vi "RT Main v0.1.vi"() -> ()   [LabVIEW 2017]
uses:
  support/Controls/All Inputs.ctl
  support/Controls/Index Details.ctl
  Controls/Auto Delays.ctl
  Global Variables/FPGA GV.vi
  <vilib>/Utility/error.llb/Error Cluster From Error Code.vi
  <vilib>/rvi/errors/niLvFpgaAdjustHostInterfaceError.vi
  Global Variables/Network Globals.vi
  Global Variables/RT GV.vi
  support/Message Queue/Enqueue Message (Single).vi
  <vilib>/FPGAPlugInAG/Dynamic/niLvFpga_Close_Dynamic.vi
  <vilib>/rvi/interface/nirviReadWriteControl/nirviReadWriteControl.xnode
  Controls/FPGA Ref.ctl
  <vilib>/rvi/interface/nirviCloseFPGA/nirviCloseFPGA.xnode
  support/Message Queue/Message Queue.lvlib
  NiFpgaLv.dll
  <vilib>/rvi/interface/Simulation/niFpgaSimulationCallBeginRW.vi
panel:
  out "error out":errorcluster
  out "Wrong Message":string
  in  "Stop Button":bool
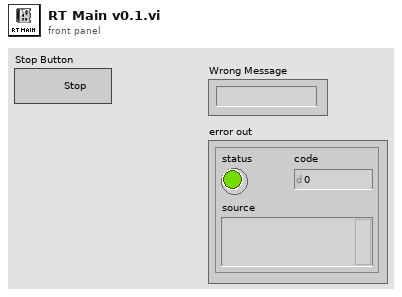
[diagram p1: front panel]
types:
  T1 = typedef "FPGA Ref.ctl" = refnum<k20>
  T2 = cluster{"TL_Red":bool, "TL_Orange":bool, "TL_Green":bool, "TL_Buzzer":bool, "SOL_Index_Rotary_CW":bool, "SOL_Index_CNVR_Rotary_CCW":bool, "SOL_Index_CNVR_Stopper_Rear":bool, "SOL_Index_CNVR_Output _Separator _Rear":bool, "Bowl  Feeder_ ON":bool, "Pump_CNVR_Motor _ON":bool, "SOL_Gating_CYL_Rear":bool, "SOL_Tube_Feed_Agitatator":bool, "SOL_Tube_Feed_Gating_CYL":bool, "SOL_Insertion _CYL":bool, "SOL_Insertion_Clamp_CYL":bool, "SOL_Cutting_CYL":bool, "SOL_Cutting_Clamp_CYL":bool, "SOL_Insertion_Air_Nozzle":bool, "SOL_Measurement_CYL":bool, "SOL_Measure_Clamp_CYL":bool, "SOL_Rejection CYL_1":bool, "SOL_Rejection CYL_2":bool, "SOL_Rejection CYL_3":bool, "SOL_Rejection CYL_4":bool, "DO1.24":bool, "DO1.25":bool, "DO1.26":bool, "DO1.27":bool, "DO1.28":bool, "DO1.29":bool, "DO1.30":bool, "DO1.31":bool}
  T3 = typedef "All Inputs.ctl" = cluster{"DI 1":cluster{"Machine_ON":bool, "E_stop ":bool, "SW_Pressure":bool, "SW_Start ":bool, "SW_Reset":bool, "SW_Stop":bool, "SW_Door":bool, "RS_Index_Rotary_CW":bool, "RS_Index_Rotary_CCW":bool, "RS_Index_Stopper _Rear":bool, "RS_Index_Output_Separator_Rear":bool, "PES_Index_Pallet_Sensor":bool, "PES_Index_Output_Part Sensor":bool, "ICS_BF_Low_Level_1":bool, "ICS_BF_Low_Level_2":bool, "ICS_BF_Pump_CNVR_Full_1":bool, "ICS_BF_Pump_CNVR_Full_2":bool, "ICS_BF_Pump_CNVR_Full_3":bool, "ICS_BF_Pump_CNVR_Full_4":bool, "PES_PC_Pump Presence_1":bool, "PES_PC_Pump Presence_2":bool, "PES_PC_Pump Presence_3":bool, "PES_PC_Pump Presence_4":bool, "RS_Gating_Rear":bool, "PES_Pump_Interference":bool, "PES_TF_Low_Level":bool, "PES_Tube Presence_1":bool, "PES_Tube Presence_2":bool, "PES_Tube Presence_3":bool, "PES_Tube Presence_4":bool, "DI1.30":bool, "DI1.31":bool}, "DI 2":cluster{"RS_Agitatator_1_Rear ":bool, "RS_Agitatator_2_Rear ":bool, "RS_Gating CYL_Rear":bool, "RS_Insertion_1_Rear":bool, "RS_Insertion_1_Front":bool, "RS_Insertion _2_Rear":bool, "RS_Insertion _2_Front":bool, "RS_Insertion _3_Rear":bool, "RS_Insertion _3_Front":bool, "RS_Insertion _4_Rear":bool, "RS_Insertion _4_Front":bool, "RS_Insertion_Clamp_Rear":bool, "RS_Cutting_Rear":bool, "RS_Cutting_Clamp _Rear":bool, "RS_Measurement_1_Rear":bool, "RS_Measurement_2_Rear":bool, "RS_Measurement_3_Rear":bool, "RS_Measurement_4_Rear":bool, "RS_Measure_Clamp_Rear":bool, "RS_Rejection_1_Rear":bool, "RS_Rejection_2_Rear":bool, "RS_Rejection_3_Rear":bool, "RS_Rejection_4_Rear":bool, "DI2.23":bool, "DI2.24":bool, "DI2.25":bool, "DI2.26":bool, "DI2.27":bool, "DI2.28":bool, "DI2.29":bool, "DI2.30":bool, "DI2.31":bool}, "IAS 1":dbl, "IAS 2":dbl, "IAS 3":dbl, "IAS 4":dbl, "DO 1":cluster{"TL_Red":bool, "TL_Orange":bool, "TL_Green":bool, "TL_Buzzer":bool, "SOL_Index_Rotary_CW":bool, "SOL_Index_CNVR_Rotary_CCW":bool, "SOL_Index_CNVR_Stopper_Rear":bool, "SOL_Index_CNVR_Output _Separator _Rear":bool, "Bowl  Feeder_ ON":bool, "Pump_CNVR_Motor _ON":bool, "SOL_Gating_CYL_Rear":bool, "SOL_Tube_Feed_Agitatator":bool, "SOL_Tube_Feed_Gating_CYL":bool, "SOL_Insertion _CYL":bool, "SOL_Insertion_Clamp_CYL":bool, "SOL_Cutting_CYL":bool, "SOL_Cutting_Clamp_CYL":bool, "SOL_Insertion_Air_Nozzle":bool, "SOL_Measurement_CYL":bool, "SOL_Measure_Clamp_CYL":bool, "SOL_Rejection CYL_1":bool, "SOL_Rejection CYL_2":bool, "SOL_Rejection CYL_3":bool, "SOL_Rejection CYL_4":bool, "DO1.24":bool, "DO1.25":bool, "DO1.26":bool, "DO1.27":bool, "DO1.28":bool, "DO1.29":bool, "DO1.30":bool, "DO1.31":bool}}
  T4 = typedef "Index Details.ctl" = cluster{"Time (ms)":u32, "Waveform Graph":i16[]}
  T5 = typedef "Auto Delays.ctl" = cluster{"TF Delays":u32[], "Insertion Delays":u32[], "Cutting Delays":u32[]}
  T6 = cluster{"Machine_ON":bool, "E_stop ":bool, "SW_Pressure":bool, "SW_Start ":bool, "SW_Reset":bool, "SW_Stop":bool, "SW_Door":bool, "RS_Index_Rotary_CW":bool, "RS_Index_Rotary_CCW":bool, "RS_Index_Stopper _Rear":bool, "RS_Index_Output_Separator_Rear":bool, "PES_Index_Pallet_Sensor":bool, "PES_Index_Output_Part Sensor":bool, "ICS_BF_Low_Level_1":bool, "ICS_BF_Low_Level_2":bool, "ICS_BF_Pump_CNVR_Full_1":bool, "ICS_BF_Pump_CNVR_Full_2":bool, "ICS_BF_Pump_CNVR_Full_3":bool, "ICS_BF_Pump_CNVR_Full_4":bool, "PES_PC_Pump Presence_1":bool, "PES_PC_Pump Presence_2":bool, "PES_PC_Pump Presence_3":bool, "PES_PC_Pump Presence_4":bool, "RS_Gating_Rear":bool, "PES_Pump_Interference":bool, "PES_TF_Low_Level":bool, "PES_Tube Presence_1":bool, "PES_Tube Presence_2":bool, "PES_Tube Presence_3":bool, "PES_Tube Presence_4":bool, "DI1.30":bool, "DI1.31":bool}
  T7 = cluster{"RS_Agitatator_1_Rear ":bool, "RS_Agitatator_2_Rear ":bool, "RS_Gating CYL_Rear":bool, "RS_Insertion_1_Rear":bool, "RS_Insertion_1_Front":bool, "RS_Insertion _2_Rear":bool, "RS_Insertion _2_Front":bool, "RS_Insertion _3_Rear":bool, "RS_Insertion _3_Front":bool, "RS_Insertion _4_Rear":bool, "RS_Insertion _4_Front":bool, "RS_Insertion_Clamp_Rear":bool, "RS_Cutting_Rear":bool, "RS_Cutting_Clamp _Rear":bool, "RS_Measurement_1_Rear":bool, "RS_Measurement_2_Rear":bool, "RS_Measurement_3_Rear":bool, "RS_Measurement_4_Rear":bool, "RS_Measure_Clamp_Rear":bool, "RS_Rejection_1_Rear":bool, "RS_Rejection_2_Rear":bool, "RS_Rejection_3_Rear":bool, "RS_Rejection_4_Rear":bool, "DI2.23":bool, "DI2.24":bool, "DI2.25":bool, "DI2.26":bool, "DI2.27":bool, "DI2.28":bool, "DI2.29":bool, "DI2.30":bool, "DI2.31":bool}
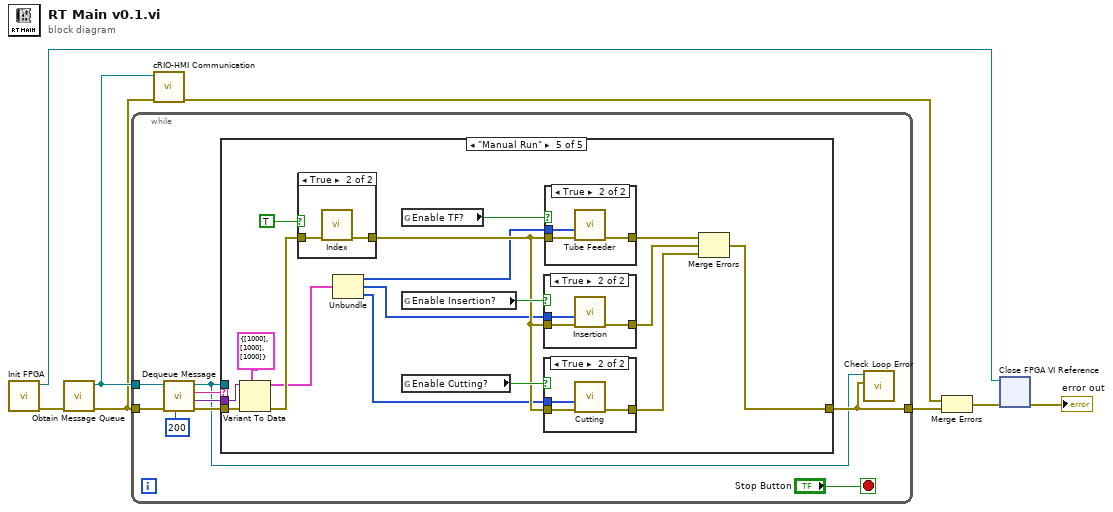
[diagram p0: block diagram]
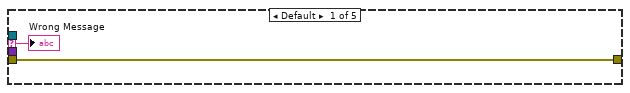
[diagram p2: hidden frame]
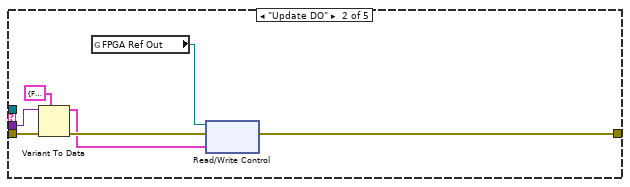
[diagram p3: hidden frame]
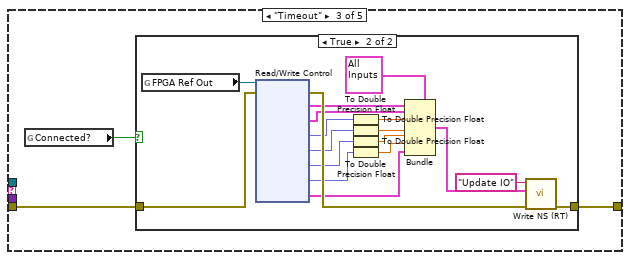
[diagram p4: hidden frame]
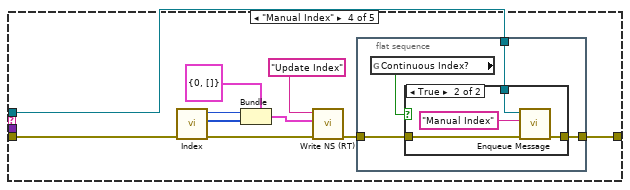
[diagram p6: hidden frame]
diagram:
  n1 = call "Init FPGA.vi"() -> ("error out"=w8:errorcluster, "FPGA Ref Out"=w2:T1)  [unwired: 10 in]
  n2 = call "Obtain Message Queue.vi"("error in (no error)"=w8) -> ("error out"=w1:errorcluster, "Message Queue"=w7:refnum<queue>)  [unwired: 9 in]
  n3 = while {
    tunnel: w1 -> [w16]
    tunnel: w7 -> [w15]
    tunnel: [w11] -> w6
    stop <- "Stop Button" stop-if-true
    n4 = call "Dequeue Message.vi"("timeout"=200, "error in (no error)"=w16, "Message Queue"=w15) -> ("error out"=w14:errorcluster, "Message Data"=w12:variant, "Message"=w13:string, "dup Message Queue"=w10:refnum<queue>)  [unwired: 5 in]
    n5 = case shown="\"Manual Run\"" w13 {
      selector: w13 -> [w19 _ _ _ _]
      tunnel: w14 -> [w18 w26 w28 w58 w75]
      tunnel: w10 -> [_ _ _ w50 _]
      tunnel: w12 -> [_ w25 _ _ w68]
      tunnel: [w18 w21 w29 w51 w76] -> w11
      frame Default {
        "Wrong Message" <- w19
      }
      frame "Update DO" {
        n6 = Variant To Data(error in=w26, type=T2 {"TL_Red"=FALSE, "TL_Orange"=FALSE, "TL_Green"=FALSE, "TL_Buzzer"=FALSE, "SOL_Index_Rotary_CW"=FALSE, "SOL_Index_CNVR_Rotary_CCW"=FALSE, "SOL_Index_CNVR_Stopper_Rear"=FALSE, "SOL_Index_CNVR_Output _Separator _Rear"=FALSE, "Bowl  Feeder_ ON"=FALSE, "Pump_CNVR_Motor _ON"=FALSE, "SOL_Gating_CYL_Rear"=FALSE, "SOL_Tube_Feed_Agitatator"=FALSE, "SOL_Tube_Feed_Gating_CYL"=FALSE, "SOL_Insertion _CYL"=FALSE, "SOL_Insertion_Clamp_CYL"=FALSE, "SOL_Cutting_CYL"=FALSE, "SOL_Cutting_Clamp_CYL"=FALSE, "SOL_Insertion_Air_Nozzle"=FALSE, "SOL_Measurement_CYL"=FALSE, "SOL_Measure_Clamp_CYL"=FALSE, "SOL_Rejection CYL_1"=FALSE, "SOL_Rejection CYL_2"=FALSE, "SOL_Rejection CYL_3"=FALSE, "SOL_Rejection CYL_4"=FALSE, "DO1.24"=FALSE, "DO1.25"=FALSE, "DO1.26"=FALSE, "DO1.27"=FALSE, "DO1.28"=FALSE, "DO1.29"=FALSE, "DO1.30"=FALSE, "DO1.31"=FALSE} ("DO 1"), Variant=w25) -> (data=w20:T2, error out=w22:errorcluster)
        n7 = global read "FPGA GV.vi" "FPGA Ref Out"() -> (w23:T1)
        n8 = xnode "Read/Write Control"("FPGA VI Reference In"=w23, "error in"=w22, "DO 1"=w20) -> ("error out"=w21:errorcluster)  [unwired: 1 out]
      }
      frame "Timeout" {
        n9 = global read "Network Globals.vi" "Connected?"() -> (w27:bool)
        n10 = case shown="True" w27 {
          tunnel: [w30 w47] -> w29
          tunnel: w28 -> [w30 w45]
          frame False {
          }
          frame True {
            n11 = global read "FPGA GV.vi" "FPGA Ref Out"() -> (w46:T1)
            n12 = xnode "Read/Write Control"("FPGA VI Reference In"=w46, "error in"=w45) -> ("error out"=w44:errorcluster, "DI 1"=w43:T6, "DI 2"=w42:T7, "AI0"=w41:fxp<+/-,27,6>, "AI1"=w36:fxp<+/-,27,6>, "AI2"=w35:fxp<+/-,27,6>, "AI3"=w34:fxp<+/-,27,6>, "DO 1"=w31:T2)  [unwired: 1 out]
            n13 = To Double Precision Float(number=w41) -> (double precision float=w40:dbl)
            n14 = To Double Precision Float(number=w36) -> (double precision float=w39:dbl)
            n15 = To Double Precision Float(number=w35) -> (double precision float=w38:dbl)
            n16 = To Double Precision Float(number=w34) -> (double precision float=w37:dbl)
            n17 = Bundle(cluster=T3 {"DI 1"={"Machine_ON"=FALSE, "E_stop "=FALSE, "SW_Pressure"=FALSE, "SW_Start "=FALSE, "SW_Reset"=FALSE, "SW_Stop"=FALSE, "SW_Door"=FALSE, "RS_Index_Rotary_CW"=FALSE, "RS_Index_Rotary_CCW"=FALSE, "RS_Index_Stopper _Rear"=FALSE, "RS_Index_Output_Separator_Rear"=FALSE, "PES_Index_Pallet_Sensor"=FALSE, "PES_Index_Output_Part Sensor"=FALSE, "ICS_BF_Low_Level_1"=FALSE, "ICS_BF_Low_Level_2"=FALSE, "ICS_BF_Pump_CNVR_Full_1"=FALSE, "ICS_BF_Pump_CNVR_Full_2"=FALSE, "ICS_BF_Pump_CNVR_Full_3"=FALSE, "ICS_BF_Pump_CNVR_Full_4"=FALSE, "PES_PC_Pump Presence_1"=FALSE, "PES_PC_Pump Presence_2"=FALSE, "PES_PC_Pump Presence_3"=FALSE, "PES_PC_Pump Presence_4"=FALSE, "RS_Gating_Rear"=FALSE, "PES_Pump_Interference"=FALSE, "PES_TF_Low_Level"=FALSE, "PES_Tube Presence_1"=FALSE, "PES_Tube Presence_2"=FALSE, "PES_Tube Presence_3"=FALSE, "PES_Tube Presence_4"=FALSE, "DI1.30"=FALSE, "DI1.31"=FALSE}, "DI 2"={"RS_Agitatator_1_Rear "=FALSE, "RS_Agitatator_2_Rear "=FALSE, "RS_Gating CYL_Rear"=FALSE, "RS_Insertion_1_Rear"=FALSE, "RS_Insertion_1_Front"=FALSE, "RS_Insertion _2_Rear"=FALSE, "RS_Insertion _2_Front"=FALSE, "RS_Insertion _3_Rear"=FALSE, "RS_Insertion _3_Front"=FALSE, "RS_Insertion _4_Rear"=FALSE, "RS_Insertion _4_Front"=FALSE, "RS_Insertion_Clamp_Rear"=FALSE, "RS_Cutting_Rear"=FALSE, "RS_Cutting_Clamp _Rear"=FALSE, "RS_Measurement_1_Rear"=FALSE, "RS_Measurement_2_Rear"=FALSE, "RS_Measurement_3_Rear"=FALSE, "RS_Measurement_4_Rear"=FALSE, "RS_Measure_Clamp_Rear"=FALSE, "RS_Rejection_1_Rear"=FALSE, "RS_Rejection_2_Rear"=FALSE, "RS_Rejection_3_Rear"=FALSE, "RS_Rejection_4_Rear"=FALSE, "DI2.23"=FALSE, "DI2.24"=FALSE, "DI2.25"=FALSE, "DI2.26"=FALSE, "DI2.27"=FALSE, "DI2.28"=FALSE, "DI2.29"=FALSE, "DI2.30"=FALSE, "DI2.31"=FALSE}, "IAS 1"=0.0, "IAS 2"=0.0, "IAS 3"=0.0, "IAS 4"=0.0, "DO 1"={"TL_Red"=FALSE, "TL_Orange"=FALSE, "TL_Green"=FALSE, "TL_Buzzer"=FALSE, "SOL_Index_Rotary_CW"=FALSE, "SOL_Index_CNVR_Rotary_CCW"=FALSE, "SOL_Index_CNVR_Stopper_Rear"=FALSE, "SOL_Index_CNVR_Output _Separator _Rear"=FALSE, "Bowl  Feeder_ ON"=FALSE, "Pump_CNVR_Motor _ON"=FALSE, "SOL_Gating_CYL_Rear"=FALSE, "SOL_Tube_Feed_Agitatator"=FALSE, "SOL_Tube_Feed_Gating_CYL"=FALSE, "SOL_Insertion _CYL"=FALSE, "SOL_Insertion_Clamp_CYL"=FALSE, "SOL_Cutting_CYL"=FALSE, "SOL_Cutting_Clamp_CYL"=FALSE, "SOL_Insertion_Air_Nozzle"=FALSE, "SOL_Measurement_CYL"=FALSE, "SOL_Measure_Clamp_CYL"=FALSE, "SOL_Rejection CYL_1"=FALSE, "SOL_Rejection CYL_2"=FALSE, "SOL_Rejection CYL_3"=FALSE, "SOL_Rejection CYL_4"=FALSE, "DO1.24"=FALSE, "DO1.25"=FALSE, "DO1.26"=FALSE, "DO1.27"=FALSE, "DO1.28"=FALSE, "DO1.29"=FALSE, "DO1.30"=FALSE, "DO1.31"=FALSE}}, "DI 1"=w43, "DI 2"=w42, "IAS 1"=w40, "IAS 2"=w39, "IAS 3"=w38, "IAS 4"=w37, "DO 1"=w31) -> (w33:T3)
            n18 = call "Write NS (RT).vi"("error in (no error)"=w44, "Message Data"=w33, "Message"="Update IO") -> ("error out"=w47:errorcluster)  [unwired: 8 in]
          }
        }
      }
      frame "Manual Index" {
        n19 = call "Index.vi"("error in (no error)"=w58) -> ("error out"=w56:errorcluster, "Waveform Graph"=w54:i16[], "Time (ms)"=w55:u32)  [unwired: 8 in]
        n20 = Bundle(cluster=T4 {"Time (ms)"=0, "Waveform Graph"=[]}, "Time (ms)"=w55, "Waveform Graph"=w54) -> (w53:T4)
        n21 = call "Write NS (RT).vi"("error in (no error)"=w56, "Message Data"=w53, "Message"="Update Index") -> ("error out"=w52:errorcluster)  [unwired: 8 in]
        n22 = flat-sequence {
          tunnel: w52 -> [w62]
          tunnel: [w61] -> w51
          tunnel: w50 -> [w59]
          frame #0 {
            n23 = global read "RT GV.vi" "Continuous Index?"() -> (w60:bool)
            n24 = case shown="True" w60 {
              tunnel: w62 -> [w63 w67]
              tunnel: [w63 w66] -> w61
              tunnel: w59 -> [_ w64]
              frame False {
              }
              frame True {
                n25 = call-poly "Enqueue Message.vi"("error in (no error)"=w67, "Message"="Manual Index", "Message Queue"=w64) -> ("error out"=w66:errorcluster)  [unwired: 7 in, 1 out]
              }
            }
          }
        }
      }
      frame "Manual Run" {
        n26 = Variant To Data(error in=w75, type=T5 {"TF Delays"=[1000], "Insertion Delays"=[1000], "Cutting Delays"=[1000]}, Variant=w68) -> (data=w72:T5, error out=w74:errorcluster)
        n27 = case shown="True" TRUE {
          tunnel: [w89 w91] -> w78
          tunnel: w74 -> [w89 w90]
          frame False {
          }
          frame True {
            n28 = call "Index.vi"("error in (no error)"=w90) -> ("error out"=w91:errorcluster)  [unwired: 8 in, 2 out]
          }
        }
        n29 = Unbundle(w72) -> ("TF Delays"=w71:u32[], "Insertion Delays"=w70:u32[], "Cutting Delays"=w69:u32[])
        n30 = global read "RT GV.vi" "Enable TF?"() -> (w79:bool)
        n31 = global read "RT GV.vi" "Enable Insertion?"() -> (w80:bool)
        n32 = global read "RT GV.vi" "Enable Cutting?"() -> (w81:bool)
        n33 = case shown="True" w80 {
          tunnel: w78 -> [w92 w95]
          tunnel: [w92 w94] -> w83
          tunnel: w70 -> [_ w93]
          frame False {
          }
          frame True {
            n34 = call "Insertion.vi"("error in (no error)"=w95, "Insertion Delays"=w93) -> ("error out"=w94:errorcluster)  [unwired: 7 in, 2 out]
          }
        }
        n35 = case shown="True" w81 {
          tunnel: w78 -> [w85 w88]
          tunnel: [w85 w87] -> w84
          tunnel: w69 -> [_ w86]
          frame False {
          }
          frame True {
            n36 = call "Cutting.vi"("error in (no error)"=w88, "Cutting Delays"=w86) -> ("error out"=w87:errorcluster)  [unwired: 8 in, 1 out]
          }
        }
        n37 = case shown="True" w79 {
          tunnel: w78 -> [w96 w99]
          tunnel: [w96 w98] -> w82
          tunnel: w71 -> [_ w97]
          frame False {
          }
          frame True {
            n38 = call "Tube Feeder.vi"("error in (no error)"=w99, "TF Delays"=w97) -> ("error out"=w98:errorcluster)  [unwired: 8 in, 1 out]
          }
        }
        n39 = Merge Errors(w82, w83, w84) -> (w76:errorcluster)
      }
    }
    n40 = call "Check Loop Error.vi"("error to process"=w11, "Message Queue"=w10) -> ()  [unwired: 8 in, 2 out]
  }
  n41 = call "cRIO-HMI Communication.vi"("error in (no error)"=w1, "Message Queue"=w7) -> ("error out"=w5:errorcluster)  [unwired: 9 in]
  n42 = Merge Errors(w5, w6) -> (w4:errorcluster)
  n43 = xnode ("Close FPGA VI Reference")("FPGA VI Reference In"=w2, "error in"=w4) -> ("error out"=→"error out":errorcluster)
